vi "PPR-simulate-dashboard.vi"() -> ()   [LabVIEW 2019]
uses:
  Diff_Drive_System/PPR_DRIVE_GLOBALS.vi
  Simulation/PPR_SIM_SIM_Globals.vi
  Trajectory Following/PPR_TRAJECTORY_GLOBALS.vi
  Vision_Interface/PPS_Vision_Globals.vi
  <vilib>/Rock Robotics/WPI/ThirdParty/MJansen/PathPlanner/PathPlanner24.lvlib
  <vilib>/Rock Robotics/WPI/ThirdParty/JAS_Junk/TrajLib/TypeDef/ROTATION2D.ctl
  <vilib>/Rock Robotics/WPI/ThirdParty/JAS_Junk/TrajLib/Trajectory_Library.lvlib
  <vilib>/Rock Robotics/WPI/ThirdParty/JAS_Junk/TrajLib/TypeDef/CHASSIS_SPEEDS.ctl
  <vilib>/Rock Robotics/WPI/ThirdParty/JAS_Junk/TrajLib/TypeDef/TRANSLATION2D.ctl
  <vilib>/Rock Robotics/WPI/ThirdParty/JAS_Junk/TrajLib/TypeDef/POSE2D.ctl
  <vilib>/Rock Robotics/WPI/ThirdParty/MJansen/PathPlanner/TypeDef/PathPlannerPathConstraints.ctl
  <vilib>/Rock Robotics/WPI/ThirdParty/MJansen/PathPlanner/TypeDef/PathPlannerTrajectoryState.ctl
  <vilib>/Rock Robotics/WPI/ThirdParty/MJansen/PathPlanner/TypeDef/PathPlannerTrajectory.ctl
panel:
  in  "Tab Control":T1(tab)
  out "Battery Voltage":dbl(graph)
  out "Drive Speed":cluster{"Motor Dmd":dbl, "Motor Dmd":dbl}(graph)
  out "Drive Motor Demands":cluster{"Motor Dmd":dbl, "Motor Dmd":dbl}(graph)
  out "GyroReading_Degreees":dbl format="%15.3f"
  out "Encoder Distances":dbl[](array[numeric]) format="%17.2f"
  out "Encoder Velocities":dbl[](array[numeric]) format="%17.2f"
  out "Motor Demands":dbl[](array[numeric]) format="%17.2f"
  out "Battery Volts":dbl format="%16.2f"
  out "Diff Module Devices":T2(array[cluster])
  out "Wheel \nSpeed Dmd":dbl[](array[numeric]) format="%17.3f"
  out "Diff Drive Motor output":T3(graph)
  out "Diff Drive Speed M/S":T4(graph)
  out "Diff Drive Speed Error  M/S":T5(graph)
  out "Closed Loop Control":bool
  out "Orientation Angle Dmd_Rad":dbl format="%17.3f"
  out "Drv Chassis Adj Velocity DmD":T6 {"vOmega" format="%10.3f"; "vY" format="%10.3f"; "vX" format="%10.3f"}
  out "GyroHeading_Radians":dbl format="%17.2f"
  out "Orientation Angle Error_Rad":dbl format="%17.3f"
  out "Orientation Correct CO":dbl format="%17.3f"
  out "Swerve Chassis Speed":T6 {"vOmega" format="%10.3f"; "vY" format="%10.3f"; "vX" format="%10.3f"}
  out "Wheel Out":dbl[](array[numeric]) format="%17.3f"
  out "Wheel \nSpeed M/S":dbl[](array[numeric]) format="%17.3f"
  out "Wheel Speed Err":dbl[](array[numeric]) format="%17.3f"
  out "Limited Wheel \nSpeed Dmd":dbl[](array[numeric]) format="%17.3f"
  out "Vision Pose":T7={"TRANSLATION"={"X"=0.0, "Y"=0.0}, "ROTATION"={"VALUE"=0.0, "COS"=1.0, "SIN"=0.0}} {"ROTATION"."SIN" format="%13.4f"; "ROTATION"."COS" format="%13.4f"; "ROTATION"."VALUE" format="%13.4f"; "TRANSLATION"."Y" format="%14.3f"; "TRANSLATION"."X" format="%14.3f"}
  out "Vision\nPose":bool
  out "Trajectory Status":T10(graph)
  out "Trajectory Execution \nClosed Loop":bool
  out "Trajectory Error":T11(graph)
  out "Traj_OnTarget":bool
  out "Traj Heading Dmd Deg":dbl format="%17.2f"
  out "Traj Final Heading Dmd Deg":dbl format="%17.2f"
  out "Traj Sample Time Sec":dbl format="%17.2f"
  out "Traj Rot Vel FF Rad/Sec":dbl format="%17.2f"
  out "Relative Trajectory Pose":T7={"TRANSLATION"={"X"=0.0, "Y"=0.0}, "ROTATION"={"VALUE"=0.0, "COS"=1.0, "SIN"=0.0}} {"ROTATION"."SIN" format="%13.4f"; "ROTATION"."COS" format="%13.4f"; "ROTATION"."VALUE" format="%13.4f"; "TRANSLATION"."Y" format="%14.3f"; "TRANSLATION"."X" format="%14.3f"}
  out "Absolute Odometry \nPose":T7={"TRANSLATION"={"X"=0.0, "Y"=0.0}, "ROTATION"={"VALUE"=0.0, "COS"=1.0, "SIN"=0.0}} {"ROTATION"."SIN" format="%13.4f"; "ROTATION"."COS" format="%13.4f"; "ROTATION"."VALUE" format="%13.4f"; "TRANSLATION"."Y" format="%14.3f"; "TRANSLATION"."X" format="%14.3f"}
  out "Other ABS Odometry\nPose":T7={"TRANSLATION"={"X"=0.0, "Y"=0.0}, "ROTATION"={"VALUE"=0.0, "COS"=1.0, "SIN"=0.0}} {"ROTATION"."SIN" format="%13.4f"; "ROTATION"."COS" format="%13.4f"; "ROTATION"."VALUE" format="%13.4f"; "TRANSLATION"."Y" format="%14.3f"; "TRANSLATION"."X" format="%14.3f"}
  out "Absolue Trajectory":cluster{dbl[], dbl[]}(graph)
  out "Absolute Trajectory":T12 {"States"."TargetHolonomicRotation"."SIN" format="%13.4f"; "States"."TargetHolonomicRotation"."COS" format="%13.4f"; "States"."TargetHolonomicRotation"."VALUE" format="%13.4f"; "States"."Heading"."SIN" format="%13.4f"; "States"."Heading"."COS" format="%13.4f"; "States"."Heading"."VALUE" format="%13.4f"; "States"."PositionMeters"."Y" format="%14.3f"; "States"."PositionMeters"."X" format="%14.3f"}
  out "Relative Trajectory":cluster{dbl[], dbl[]}(graph)
  # "SIMULATION"
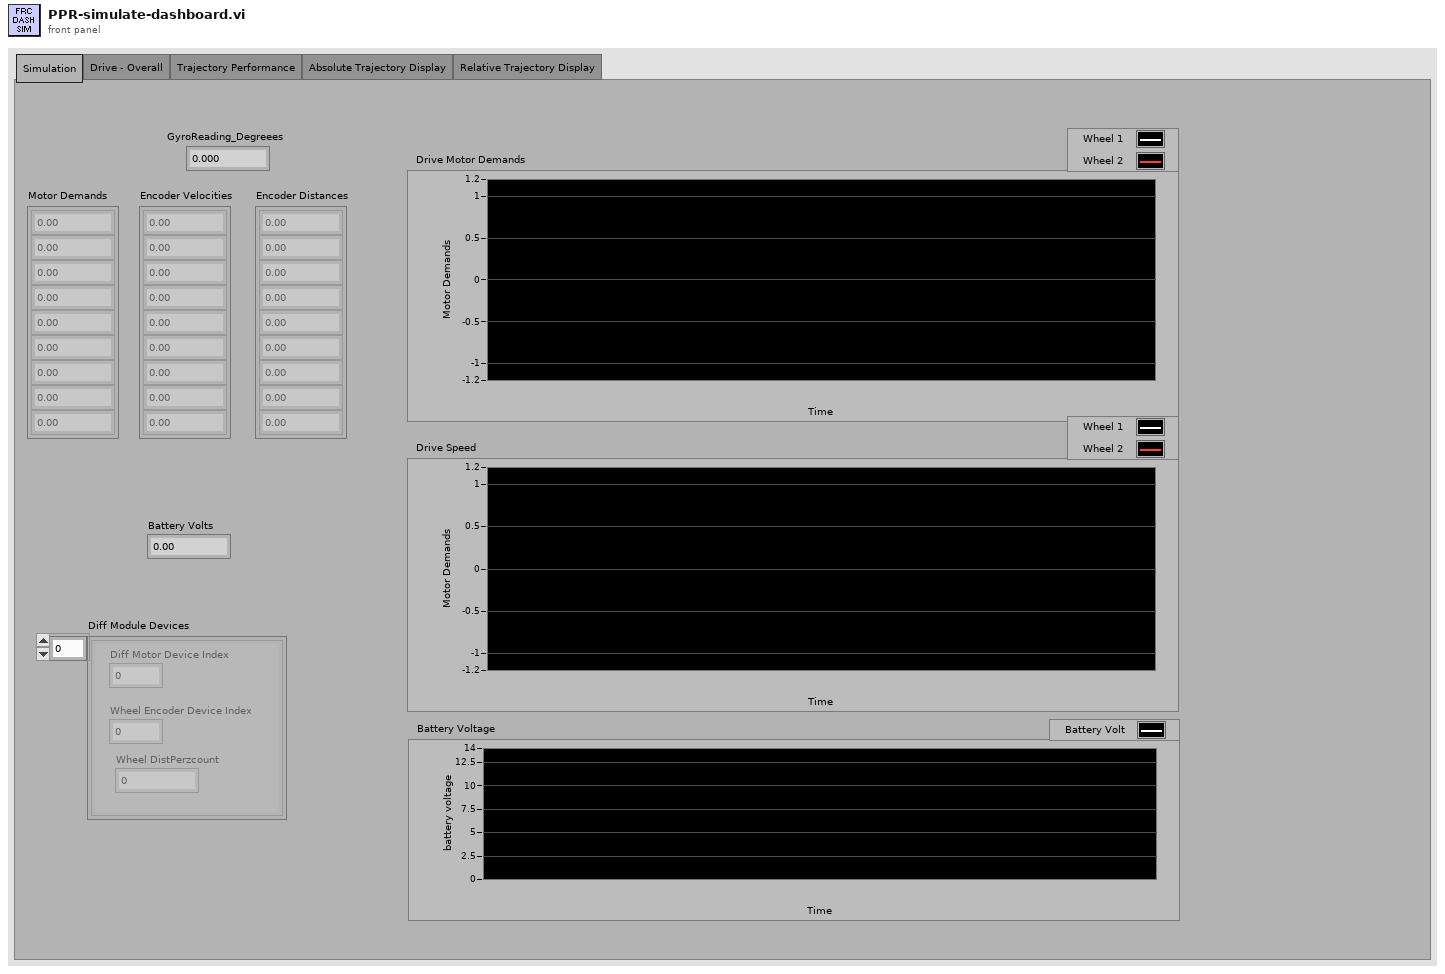
[diagram p1: front panel]
types:
  T1 = enum32{"Simulation", "Drive - Overall", "Trajectory Performance", "Absolute Trajectory Display", "Relative Trajectory Display"}
  T2 = cluster{"Diff Motor Device Index":i32, "Wheel Encoder Device Index":i32, "Wheel DistPerzcount":dbl}[]
  T3 = cluster{"Left Wheel Motor Out":dbl, "Right Wheel Motor Out":dbl}
  T4 = cluster{"Left Wheel Speed M/S":dbl, "Right Wheel Speed M/S":dbl}
  T5 = cluster{"Left Wheel Speed Err M/S":dbl, "Right Wheel Speed Err M/S":dbl}
  T6 = typedef "Trajectory_Library.lvlib/CHASSIS_SPEEDS.ctl" = cluster{"vX":dbl, "vY":dbl, "vOmega":dbl}
  T7 = typedef "Trajectory_Library.lvlib/POSE2D.ctl" = cluster{"TRANSLATION":T8, "ROTATION":T9}
  T8 = typedef "Trajectory_Library.lvlib/TRANSLATION2D.ctl" = cluster{"X":dbl, "Y":dbl}
  T9 = typedef "Trajectory_Library.lvlib/ROTATION2D.ctl" = cluster{"VALUE":dbl, "COS":dbl, "SIN":dbl}
  T10 = cluster{dbl, dbl, dbl, "Traj_Sample_Time_Sec":dbl}
  T11 = cluster{"Traj X Err":dbl, "Traj Y Err":dbl, "Traj Heading Err":dbl}
  T12 = typedef "PathPlanner24.lvlib/PathPlannerTrajectory.ctl" = cluster{"States":T13[]}
  T13 = typedef "PathPlanner24.lvlib/PathPlannerTrajectoryState.ctl" = cluster{"TimeSeconds":dbl, "VelocityMPS":dbl, "AccerationMpsSq":dbl, "HeadingAngularVelRadPerSec":dbl, "PositionMeters":T8, "Heading":T9, "TargetHolonomicRotation":T9, "CurvatureRadPerMeter":dbl, "PathPlannerConstraints":T14, "DeltaPos":dbl}
  T14 = typedef "PathPlanner24.lvlib/PathPlannerPathConstraints.ctl" = cluster{"MaxVelocityMps;":dbl, "MaxAccelerationMpsSq;":dbl, "MaxAngularVelRadPsEc;":dbl, "MaxAngularAccRadPSecSq":dbl, "Exists":bool}
  T15 = cluster{"Traj X Err_FT":dbl, "Traj Y Err_FT":dbl, "Traj Heading Err_DEG":dbl}
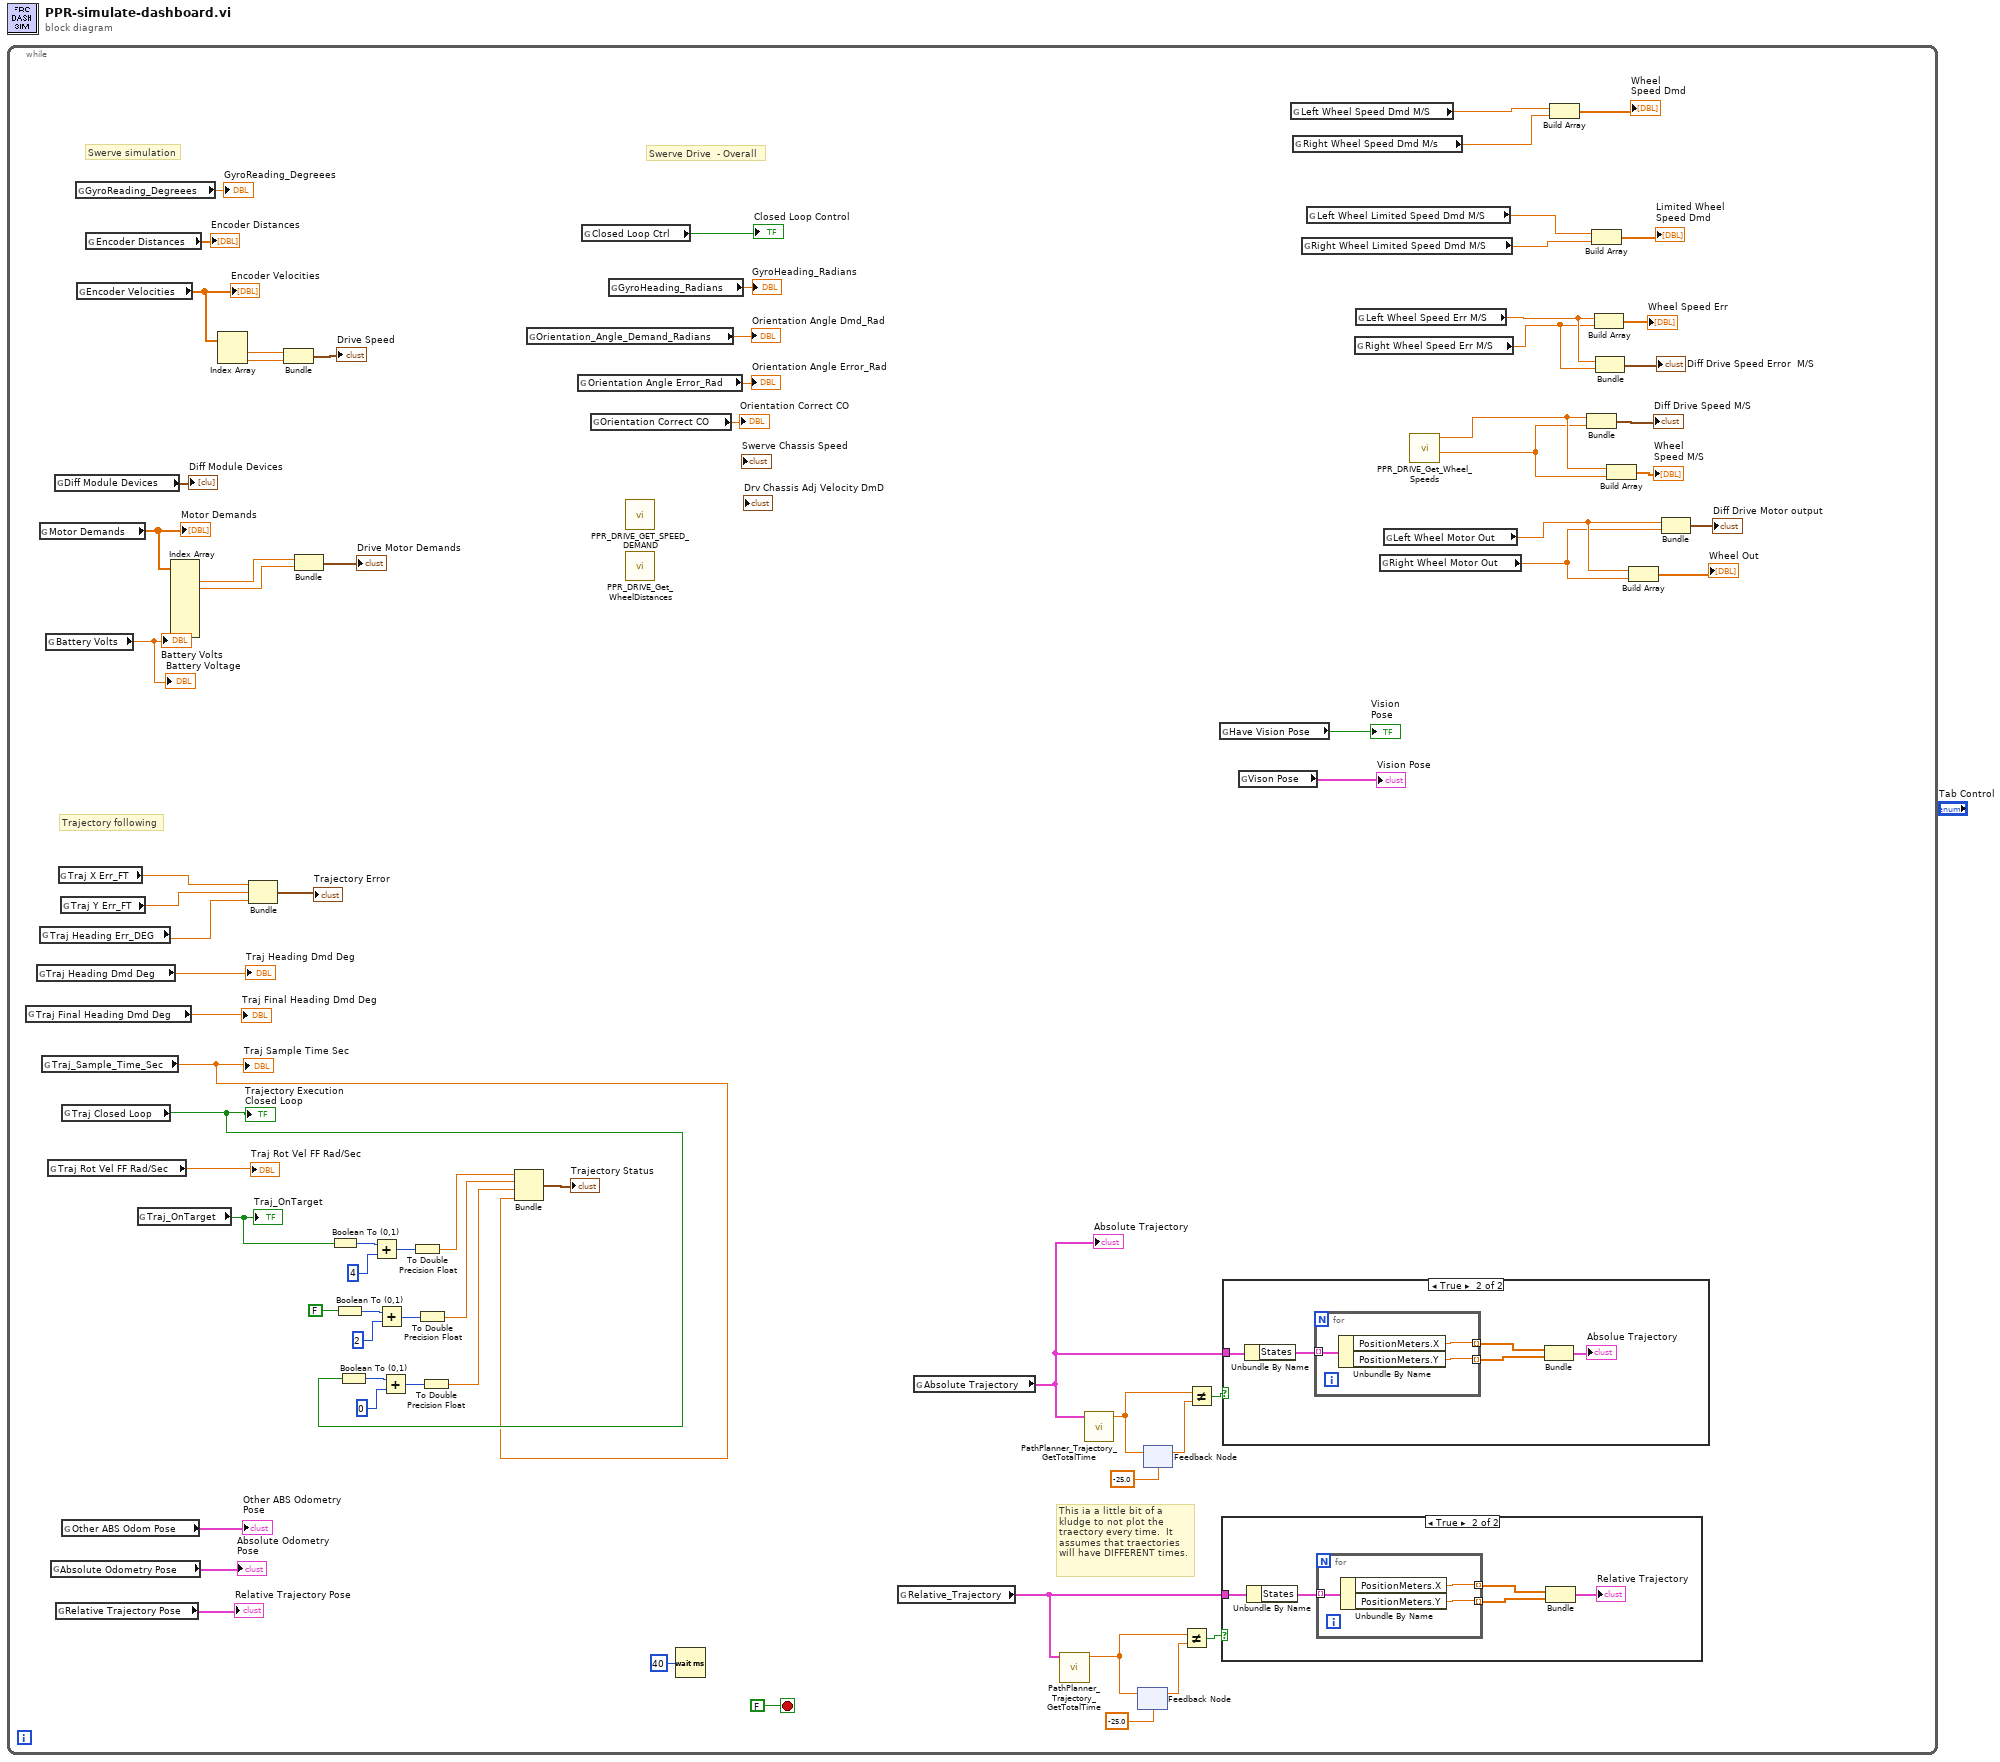
[diagram p0: block diagram]
diagram:
  n1 = while {
    stop <- FALSE stop-if-true
    # "This ia a little bit of a \nkludge to not plot the\ntraectory every time.  It \nassumes that traectories\nwill have DIFFERENT times."
    # "Trajectory following"
    # "Swerve simulation"
    # "Swerve Drive  - Overall"
    n2 = global read "PPR_TRAJECTORY_GLOBALS.vi" "Traj Final Heading Dmd Deg"() -> (→"Traj Final Heading Dmd Deg":dbl)
    n3 = global read "PPR_TRAJECTORY_GLOBALS.vi" "Traj Heading Dmd Deg"() -> (→"Traj Heading Dmd Deg":dbl)
    n4 = global read "PPR_SIM_SIM_Globals.vi" "Motor Demands"() -> (w67:dbl[])
    "Motor Demands" <- w67
    n5 = global read "PPR_TRAJECTORY_GLOBALS.vi" "Traj Heading Err_DEG"() -> (w62:dbl)
    n6 = global read "PPR_TRAJECTORY_GLOBALS.vi" "Traj_Sample_Time_Sec"() -> (w43:dbl)
    "Traj Sample Time Sec" <- w43
    n7 = global read "PPR_SIM_SIM_Globals.vi" "Battery Volts"() -> (→"Battery Volts" →"Battery Voltage":dbl)
    n8 = global read "PPR_TRAJECTORY_GLOBALS.vi" "Traj Rot Vel FF Rad/Sec"() -> (→"Traj Rot Vel FF Rad/Sec":dbl)
    n9 = global read "PPR_TRAJECTORY_GLOBALS.vi" "Absolute Odometry Pose"() -> (→"Absolute Odometry \nPose":T7)
    n10 = global read "PPR_SIM_SIM_Globals.vi" "Diff Module Devices"() -> (→"Diff Module Devices":T2)
    n11 = global read "PPR_TRAJECTORY_GLOBALS.vi" "Relative Trajectory Pose"() -> (→"Relative Trajectory Pose":T7)
    n12 = global read "PPR_TRAJECTORY_GLOBALS.vi" "Traj X Err_FT"() -> (w64:dbl)
    n13 = global read "PPR_TRAJECTORY_GLOBALS.vi" "Traj Y Err_FT"() -> (w63:dbl)
    n14 = global read "PPR_TRAJECTORY_GLOBALS.vi" "Traj Closed Loop"() -> (w45:bool)
    "Trajectory Execution \nClosed Loop" <- w45
    n15 = global read "PPR_TRAJECTORY_GLOBALS.vi" "Other ABS Odom Pose"() -> (→"Other ABS Odometry\nPose":T7)
    n16 = global read "PPR_SIM_SIM_Globals.vi" "GyroReading_Degreees"() -> (→"GyroReading_Degreees":dbl)
    n17 = global read "PPR_SIM_SIM_Globals.vi" "Encoder Velocities"() -> (w4:dbl[])
    "Encoder Velocities" <- w4
    n18 = global read "PPR_SIM_SIM_Globals.vi" "Encoder Distances"() -> (→"Encoder Distances":dbl[])
    n19 = global read "PPR_TRAJECTORY_GLOBALS.vi" "Traj_OnTarget"() -> (w57:bool)
    "Traj_OnTarget" <- w57
    n20 = Index Array(array=w67) -> (element #1=w66:dbl, element #2=w5:dbl)  [unwired: 8 in, 6 out]
    n21 = Index Array(array=w4) -> (element #1=w3:dbl, element #2=w2:dbl)  [unwired: 2 in]
    n22 = Bundle("Traj X Err_FT"=w64, "Traj Y Err_FT"=w63, "Traj Heading Err_DEG"=w62) -> (→"Trajectory Error":T15)  [unwired: 1 in]
    n23 = Bundle("Motor Dmd"=w3, "Motor Dmd"=w2) -> (→"Drive Speed":cluster{"Motor Dmd":dbl, "Motor Dmd":dbl})  [unwired: 1 in]
    n24 = Bundle("Motor Dmd"=w66, "Motor Dmd"=w5) -> (→"Drive Motor Demands":cluster{"Motor Dmd":dbl, "Motor Dmd":dbl})  [unwired: 1 in]
    n25 = Boolean To (0,1)(Boolean=w57) -> (0, 1=w55:i16)
    n26 = Boolean To (0,1)(Boolean=FALSE) -> (0, 1=w52:i16)
    n27 = Boolean To (0,1)(Boolean=w45) -> (0, 1=w48:i16)
    n28 = Add(x=w55, y=i16 4) -> (x+y=w54:i16)
    n29 = Add(x=w52, y=i16 2) -> (x+y=w51:i16)
    n30 = Add(x=w48, y=i16 0) -> (x+y=w47:i16)
    n31 = To Double Precision Float(number=w54) -> (double precision float=w56:dbl)
    n32 = To Double Precision Float(number=w51) -> (double precision float=w49:dbl)
    n33 = To Double Precision Float(number=w47) -> (double precision float=w44:dbl)
    n34 = Bundle(w56, w49, w44, "Traj_Sample_Time_Sec"=w43) -> (→"Trajectory Status":T10)  [unwired: 1 in]
    n35 = global read "PPR_DRIVE_GLOBALS.vi" "Orientation_Angle_Demand_Radians"() -> (→"Orientation Angle Dmd_Rad":dbl)
    n36 = global read "PPR_DRIVE_GLOBALS.vi" "Orientation Angle Error_Rad"() -> (→"Orientation Angle Error_Rad":dbl)
    n37 = global read "PPR_DRIVE_GLOBALS.vi" "Closed Loop Ctrl"() -> (→"Closed Loop Control":bool)
    n38 = global read "PPR_DRIVE_GLOBALS.vi" "Orientation Correct CO"() -> (→"Orientation Correct CO":dbl)
    n39 = global read "PPR_DRIVE_GLOBALS.vi" "GyroHeading_Radians"() -> (→"GyroHeading_Radians":dbl)
    n40 = call "PPR_DRIVE_GET_SPEED_DEMAND.vi"() -> ()  [unwired: 10 in, 2 out]
    n41 = call "PPR_DRIVE_Get_WheelDistances.vi"() -> ()  [unwired: 10 in, 2 out]
    n42 = Wait (ms)(milliseconds to wait=u32 40) -> ()  [unwired: 1 out]
    n43 = global read "PPR_TRAJECTORY_GLOBALS.vi" "Relative_Trajectory"() -> (w25:T12)
    n44 = global read "PPR_TRAJECTORY_GLOBALS.vi" "Absolute Trajectory"() -> (w27:T12)
    "Absolute Trajectory" <- w27
    n45 = call <vilib>:"PathPlanner_Trajectory_GetTotalTime.vi"("PathPlannerTrajectory"=w25) -> ("TotalTimeSeconds"=w24:dbl)  [unwired: 10 in]
    n46 = call <vilib>:"PathPlanner_Trajectory_GetTotalTime.vi"("PathPlannerTrajectory"=w27) -> ("TotalTimeSeconds"=w26:dbl)  [unwired: 10 in]
    n47 = feedback #1(-25.0 ("TotalTime_Sec")) -> (w29:dbl)
    n48 = feedback-in #1(w24) -> ()
    n49 = feedback #2(-25.0 ("TotalTime_Sec")) -> (w32:dbl)
    n50 = feedback-in #2(w26) -> ()
    n51 = Not Equal?(x=w24, y=w29) -> (x != y?=w28:bool)
    n52 = Not Equal?(x=w26, y=w32) -> (x != y?=w31:bool)
    n53 = global read "PPS_Vision_Globals.vi" "Have Vision Pose"() -> (→"Vision\nPose":bool)
    n54 = case shown="True" w28 {
      tunnel: w25 -> [_ w78]
      frame False {
      }
      frame True {
        n55 = Unbundle By Name(w78) -> ("States"=w79:T13[])
        n56 = for {
          tunnel: [w84] -> w80 mode=indexing
          tunnel: [w83] -> w81 mode=indexing
          tunnel: w79 -> [w82] mode=indexing
          n57 = Unbundle By Name(w82) -> ("PositionMeters.X"=w84:dbl, "PositionMeters.Y"=w83:dbl)
        }
        n58 = Bundle(w80, w81) -> (→"Relative Trajectory":cluster{dbl[], dbl[]})  [unwired: 1 in]
      }
    }
    n59 = case shown="True" w31 {
      tunnel: w27 -> [_ w85]
      frame False {
      }
      frame True {
        n60 = Unbundle By Name(w85) -> ("States"=w87:T13[])
        n61 = for {
          tunnel: [w92] -> w88 mode=indexing
          tunnel: [w91] -> w89 mode=indexing
          tunnel: w87 -> [w90] mode=indexing
          n62 = Unbundle By Name(w90) -> ("PositionMeters.X"=w92:dbl, "PositionMeters.Y"=w91:dbl)
        }
        n63 = Bundle(w88, w89) -> (→"Absolue Trajectory":cluster{dbl[], dbl[]})  [unwired: 1 in]
      }
    }
    n64 = global read "PPS_Vision_Globals.vi" "Vison Pose"() -> (→"Vision Pose":T7)
    n65 = global read "PPR_DRIVE_GLOBALS.vi" "Left Wheel Speed Dmd M/S"() -> (w10:dbl)
    n66 = global read "PPR_DRIVE_GLOBALS.vi" "Right Wheel Speed Dmd M/s"() -> (w9:dbl)
    n67 = global read "PPR_DRIVE_GLOBALS.vi" "Right Wheel Limited Speed Dmd M/S"() -> (w6:dbl)
    n68 = global read "PPR_DRIVE_GLOBALS.vi" "Left Wheel Limited Speed Dmd M/S"() -> (w7:dbl)
    n69 = global read "PPR_DRIVE_GLOBALS.vi" "Right Wheel Speed Err M/S"() -> (w12:dbl)
    n70 = global read "PPR_DRIVE_GLOBALS.vi" "Left Wheel Speed Err M/S"() -> (w13:dbl)
    n71 = global read "PPR_DRIVE_GLOBALS.vi" "Right Wheel Motor Out"() -> (w18:dbl)
    n72 = global read "PPR_DRIVE_GLOBALS.vi" "Left Wheel Motor Out"() -> (w19:dbl)
    n73 = call "PPR_DRIVE_Get_Wheel_Speeds.vi"() -> ("Right Wheel Speed M/S"=w15:dbl, "Left Wheel Speed M/S"=w16:dbl)  [unwired: 10 in]
    n74 = Build Array(w10, w9) -> (→"Wheel \nSpeed Dmd":dbl[])
    n75 = Bundle("Left Wheel Speed M/S"=w16, "Right Wheel Speed M/S"=w15) -> (→"Diff Drive Speed M/S":T4)  [unwired: 1 in]
    n76 = Build Array(w7, w6) -> (→"Limited Wheel \nSpeed Dmd":dbl[])
    n77 = Build Array(w13, w12) -> (→"Wheel Speed Err":dbl[])
    n78 = Bundle("Left Wheel Speed Err M/S"=w13, "Right Wheel Speed Err M/S"=w12) -> (→"Diff Drive Speed Error  M/S":T5)  [unwired: 1 in]
    n79 = Build Array(w16, w15) -> (→"Wheel \nSpeed M/S":dbl[])
    n80 = Build Array(w19, w18) -> (→"Wheel Out":dbl[])
    n81 = Bundle("Left Wheel Motor Out"=w19, "Right Wheel Motor Out"=w18) -> (→"Diff Drive Motor output":T3)  [unwired: 1 in]
  }
